vi "Read from COM Port.vi"(8 "error in":errorcluster caption="error IO", 10 "Byte to Read (-1:All)":i32, 11 "VISA resource name in":refnum<visa-resource-name>) -> (0 "error out":errorcluster, 1 "readed Bytes":u32, 2 "String (output)":string, 3 "VISA resource name out":refnum<visa-resource-name>)   [LabVIEW 2018, in "JULABO DeviceDriver.lvlib"]
uses:
  JULABO DeviceDriver.lvlib
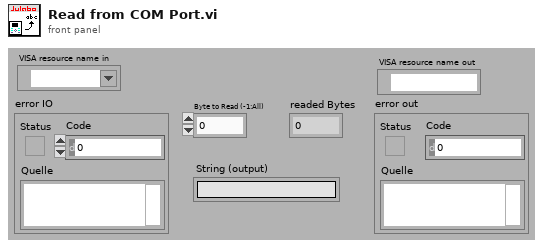
[diagram p1: front panel]
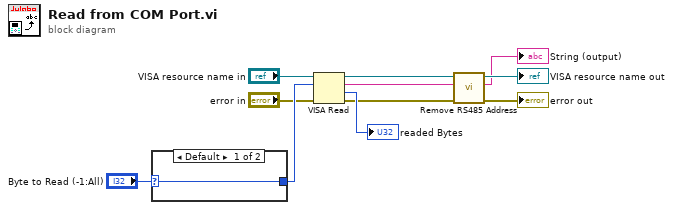
[diagram p0: block diagram]
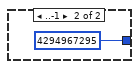
[diagram p2: hidden frame]
diagram:
  n1 = case shown="Default" "Byte to Read (-1:All)" {
    selector: "Byte to Read (-1:All)" -> [w12 _]
    tunnel: [w12 u32 4294967295 ("Anzahl der Bytes")] -> w3
    frame Default {
    }
    frame ..-1 {
    }
  }
  n2 = VISA Read(VISA resource name="VISA resource name in", byte count=w3, error in (no error)="error in") -> (VISA resource name out=w9:refnum<visa-resource-name>, read buffer=w4:string, return count=→"readed Bytes":u32, error out=w8:errorcluster)
  n3 = call "Remove RS485 Address.vi"("error in"=w8, "Command (input)"=w4, "VISA resource name in"=w9) -> ("error out"=→"error out":errorcluster, "Command (output)"=→"String (output)":string, "VISA resource name out"=→"VISA resource name out":refnum<visa-resource-name>)  [unwired: 2 in]
